vi "set-angle-to-z-axis-cord.vi"() -> ()   [LabVIEW 2013]
panel:
  in  "Axis":cluster{"X":sgl, "Y":sgl, "Z":sgl}={"X"=0.0, "Y"=0.0, "Z"=-1.0}
  out "数值输入控件":dbl
  in  "Degree":dbl
  in  "正Z轴?":bool
  # "z轴指向自己,逆时针为正角度"
  # "范围是 [ -360, 360 )"
  # "输入的是: 获取角度给的值"
  # "输出对应 正z 或 负z 轴的角度"
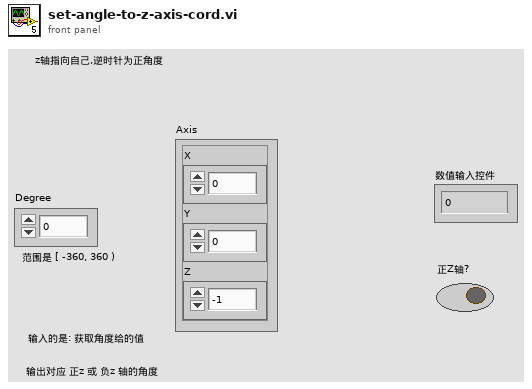
[diagram p1: front panel]
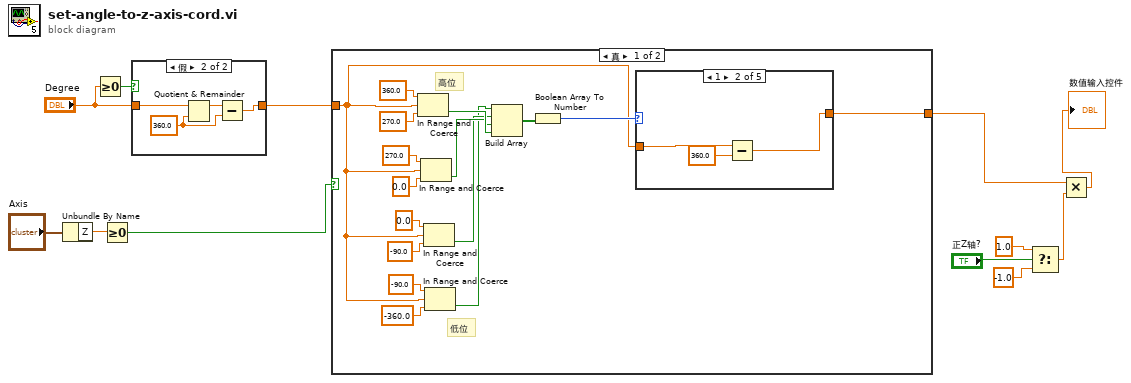
[diagram p0: block diagram]
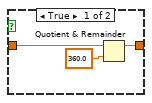
[diagram p2: hidden frame]
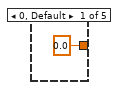
[diagram p3: hidden frame]
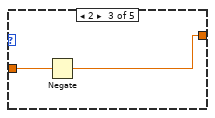
[diagram p4: hidden frame]
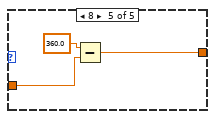
[diagram p6: hidden frame]
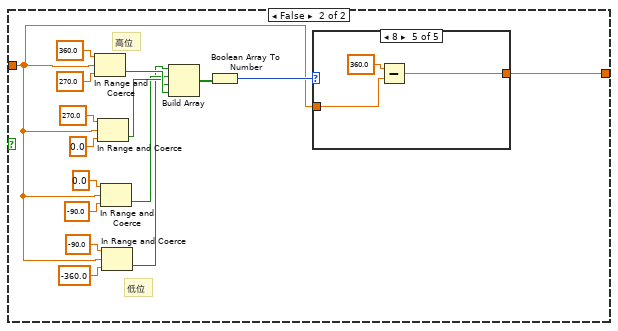
[diagram p7: hidden frame]
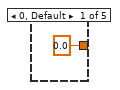
[diagram p8: hidden frame]
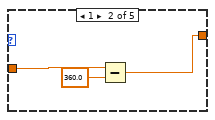
[diagram p9: hidden frame]
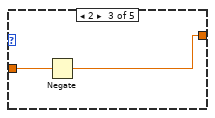
[diagram p10: hidden frame]
diagram:
  n1 = Unbundle By Name("Axis") -> ("Z"=w8:sgl)
  n2 = Greater Or Equal To 0?(x="Degree") -> (x >= 0?=w10:bool)
  n3 = Greater Or Equal To 0?(x=w8) -> (x >= 0?=w7:bool)
  n4 = case shown="假" w10 {
    tunnel: [w14 w18] -> w12
    tunnel: "Degree" -> [w13 w19]
    frame True {
      n5 = Quotient & Remainder(x=w13, y=360.0) -> (x-y*floor(x/y)=w14:dbl)  [unwired: 1 out]
    }
    frame False {
      w16 = 360.0 ("y")
      n6 = Quotient & Remainder(x=w19, y=w16) -> (x-y*floor(x/y)=w17:dbl)  [unwired: 1 out]
      n7 = Subtract(x=w17, y=w16) -> (x-y=w18:dbl)
    }
  }
  n8 = case shown="真" w7 {
    tunnel: w12 -> [w21 w47]
    tunnel: [w20 w46] -> w3
    frame True {
      # "低位"
      # "高位"
      n9 = In Range and Coerce(upper limit=360.0 ("上限"), x=w21, lower limit=270.0 ("下限")) -> (In Range?=w26:bool)  [unwired: 1 out]
      n10 = In Range and Coerce(upper limit=270.0 ("上限"), x=w21, lower limit=0.0 ("下限")) -> (In Range?=w25:bool)  [unwired: 1 out]
      n11 = In Range and Coerce(upper limit=0.0 ("上限"), x=w21, lower limit=-90.0 ("下限")) -> (In Range?=w24:bool)  [unwired: 1 out]
      n12 = In Range and Coerce(upper limit=-90.0 ("上限"), x=w21, lower limit=-360.0 ("下限")) -> (In Range?=w23:bool)  [unwired: 1 out]
      n13 = Build Array(w23, w24, w25, w26) -> (w27:bool[])
      n14 = Boolean Array To Number(Boolean array=w27) -> (number=w22:u32)
      n15 = case shown="1" w22 {
        tunnel: w21 -> [_ w39 w41 w42 w44]
        tunnel: [0.0 w37 w40 w42 w43] -> w20
        frame 0, Default {
        }
        frame 1 {
          n16 = Subtract(x=w39, y=360.0) -> (x-y=w37:dbl)
        }
        frame 2 {
          n17 = Negate(x=w41) -> (-x=w40:dbl)
        }
        frame 4 {
        }
        frame 8 {
          n18 = Subtract(x=360.0, y=w44) -> (x-y=w43:dbl)
        }
      }
    }
    frame False {
      # "低位"
      # "高位"
      n19 = In Range and Coerce(upper limit=360.0 ("上限"), x=w47, lower limit=270.0 ("下限")) -> (In Range?=w52:bool)  [unwired: 1 out]
      n20 = In Range and Coerce(upper limit=270.0 ("上限"), x=w47, lower limit=0.0 ("下限")) -> (In Range?=w51:bool)  [unwired: 1 out]
      n21 = In Range and Coerce(upper limit=0.0 ("上限"), x=w47, lower limit=-90.0 ("下限")) -> (In Range?=w50:bool)  [unwired: 1 out]
      n22 = In Range and Coerce(upper limit=-90.0 ("上限"), x=w47, lower limit=-360.0 ("下限")) -> (In Range?=w49:bool)  [unwired: 1 out]
      n23 = Build Array(w49, w50, w51, w52) -> (w53:bool[])
      n24 = Boolean Array To Number(Boolean array=w53) -> (number=w48:u32)
      n25 = case shown="8" w48 {
        tunnel: w47 -> [_ w65 w67 w68 w70]
        tunnel: [0.0 w63 w66 w68 w69] -> w46
        frame 0, Default {
        }
        frame 1 {
          n26 = Subtract(x=w65, y=360.0) -> (x-y=w63:dbl)
        }
        frame 2 {
          n27 = Negate(x=w67) -> (-x=w66:dbl)
        }
        frame 4 {
        }
        frame 8 {
          n28 = Subtract(x=360.0, y=w70) -> (x-y=w69:dbl)
        }
      }
    }
  }
  n29 = Select(t=1.0, s="正Z轴?", f=-1.0) -> (s? t:f=w2:dbl)
  n30 = Multiply(x=w3, y=w2) -> (x*y=→"数值输入控件":dbl)
